vi "disk_writeFormattedData.vi"(8 "error in":errorcluster, 10 "xml":string, 11 "DiskTemplate in":T1={"XMLRef"=[refnum, refnum, refnum, refnum, refnum, refnum], "ZipPath"=path "", "MetaFile"={"Ref"=refnum, "NextRow"=0, "NextPosition"=0, "Block"=[]}, "TempFolder"=path ""}) -> (0 "error out":errorcluster, 3 "DiskTemplate out":T1)   [LabVIEW 2020, in "NI_ExcelFile.lvlib"]
uses:
  <vilib>/express/express shared/NI_ExcelFile/NI_ExcelFile.lvlib
  <vilib>/express/express shared/NI_ExcelFile/Ctrls/disk_TemplateFile.ctl
  <vilib>/express/express shared/NI_ExcelFile/Ctrls/meta_file.ctl
  <vilib>/express/express shared/NI_ExcelFile/Ctrls/meta_Block.ctl
  <vilib>/express/express shared/NI_ExcelFile/Ctrls/meta_BlockType.ctl
  <vilib>/express/express shared/NI_ExcelFile/Ctrls/TemplateEnum.ctl
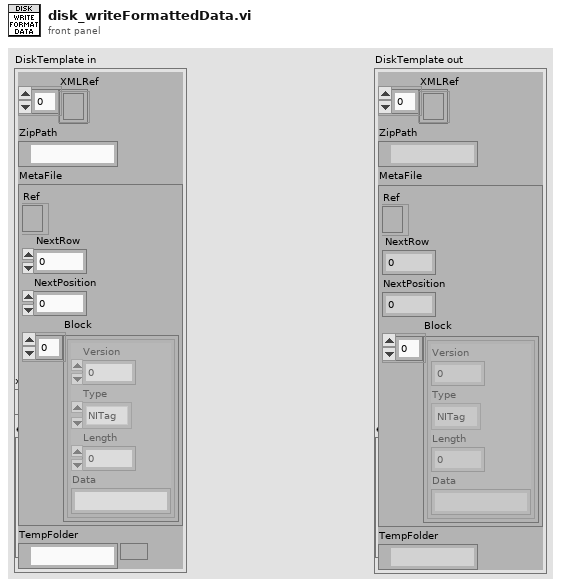
[diagram p1: front panel]
types:
  T1 = typedef "NI_ExcelFile.lvlib/disk_TemplateFile.ctl" = cluster{"XMLRef":refnum<file>[], "ZipPath":path, "MetaFile":T2, "TempFolder":path}
  T2 = typedef "NI_ExcelFile.lvlib/meta_file.ctl" = cluster{"Ref":refnum<file>, "NextRow":i32, "NextPosition":i64, "Block":T3[]}
  T3 = typedef "NI_ExcelFile.lvlib/meta_Block.ctl" = cluster{"Version":u16, "Type":T4, "Length":i32, "Data":string}
  T4 = typedef "NI_ExcelFile.lvlib/meta_BlockType.ctl" = enum16{"NITag", "File", "Column"}
  T5 = typedef "NI_ExcelFile.lvlib/TemplateEnum.ctl" = enum16{"[Content_Types].xml", ".rels", "workbook.xml", "styles.xml", "workbook.xml.rels", "sheet.xml", "app.xml", "core.xml"}
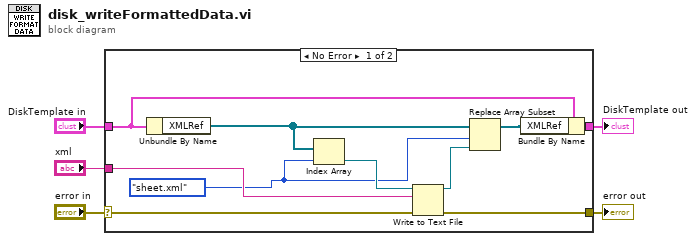
[diagram p0: block diagram]
diagram:
  n1 = case shown="No Error" "error in" {
    selector: "error in" -> [w6 w17]
    tunnel: [w14 w17] -> w5
    tunnel: "xml" -> [w13 _]
    tunnel: [w10 w16] -> w3
    tunnel: "DiskTemplate in" -> [w9 w16]
    frame No Error {
      w7 = TemplateEnum."sheet.xml" ("Template")
      n2 = Unbundle By Name(w9) -> ("XMLRef"=w11:refnum<file>[])
      n3 = Index Array(array=w11, index=w7) -> (element=w15:refnum<file>)
      n4 = Write to Text File(file (use dialog)=w15, text=w13, error in=w6) -> (refnum out=w12:refnum<file>, error out=w14:errorcluster)  [unwired: 1 in, 1 out]
      n5 = Replace Array Subset(array=w11, new element=w12, index=w7) -> (w8:refnum<file>[])
      n6 = Bundle By Name(cluster=w9, "XMLRef"=w8) -> (w10:T1)
    }
    frame Error {
    }
  }
  "error out" <- w5
  "DiskTemplate out" <- w3
